vi "Disabled.vi"(7 "Robot Mode":T2, 10 "Match Info":T1={"Autonomous Elapsed Seconds"=0.0, "TeleOp Elapsed Seconds"=0.0, "Disabled Elapsed Seconds"=0.0, "Visited Autonomous"=FALSE, "Visited TeleOp"=FALSE, "Visited Disabled"=FALSE, "Autonomous Settings"={"Autonomous Style"=enum."Independent", "VI Refnum"=refnum}}, 11 "Call Context":T3) -> ()   [LabVIEW 2015]
doc: "This VI is called each time a disabled packet is received from the DS. It is often used to prepare for the next robot mode, to calibrate sensors, etc."
uses:
  <vilib>/Rock Robotics/WPI/DriverStation/WPI_DriverStationDerivedRobotMode.ctl
  <vilib>/Rock Robotics/WPI/DriverStation/WPI_DriverStationRobotMode2.ctl
  <vilib>/Rock Robotics/WPI/DriverStation/WPI_DriverStationMatch Info.ctl
  <vilib>/Rock Robotics/WPI/Utilities/WPI_GetSetVariantRefNum.vi
  Robot Global Data.vi
  Moose Code/Auto_Conf.vi
  <vilib>/Rock Robotics/Network Tables/NT Write Boolean.vi
  <vilib>/Rock Robotics/Network Tables/NT Write Number.vi
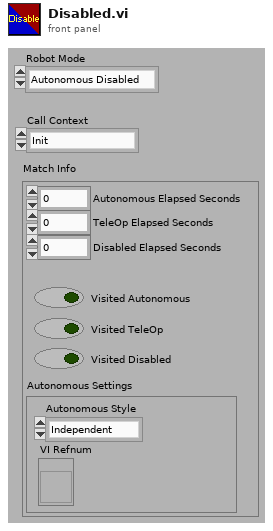
[diagram p1: front panel]
types:
  T1 = typedef "WPI_DriverStationMatch Info.ctl" = cluster{"Autonomous Elapsed Seconds":dbl, "TeleOp Elapsed Seconds":dbl, "Disabled Elapsed Seconds":dbl, "Visited Autonomous":bool, "Visited TeleOp":bool, "Visited Disabled":bool, "Autonomous Settings":cluster{"Autonomous Style":enum16{"Iterative", "Independent"}, "VI Refnum":refnum<vi>}}
  T2 = typedef "WPI_DriverStationRobotMode2.ctl" = enum16{"Autonomous Disabled", "Autonomous Enabled", "Teleop Disabled", "Teleop Enabled", "Disconnected", "Finish", "Test Disabled", "Test Enabled", "Emergency Stopped"}
  T3 = typedef "WPI_DriverStationDerivedRobotMode.ctl" = enum16{"Init", "Execute", "Stop"}
  T4 = typedef "WPI_JoystickDevRef.ctl" = cluster{"Device":T5}
  T5 = typedef "WPI_JoystickDeviceEnum.ctl" = enum16{"USB 0", "USB 1", "USB 2", "USB 3", "USB 4", "USB 5"}
  T6 = cluster{"TopLeft":bool, "TopCenter":bool, "TopRight":bool, "MiddleRight":bool, "MiddleLeft":bool, "MiddleCenter":bool, "BottomRight":bool, "BottomLeft":bool, "BottomCenter":bool, "Top":bool, "Middle":bool, "Bottom":bool, "Left":bool, "Center":bool, "Right":bool}
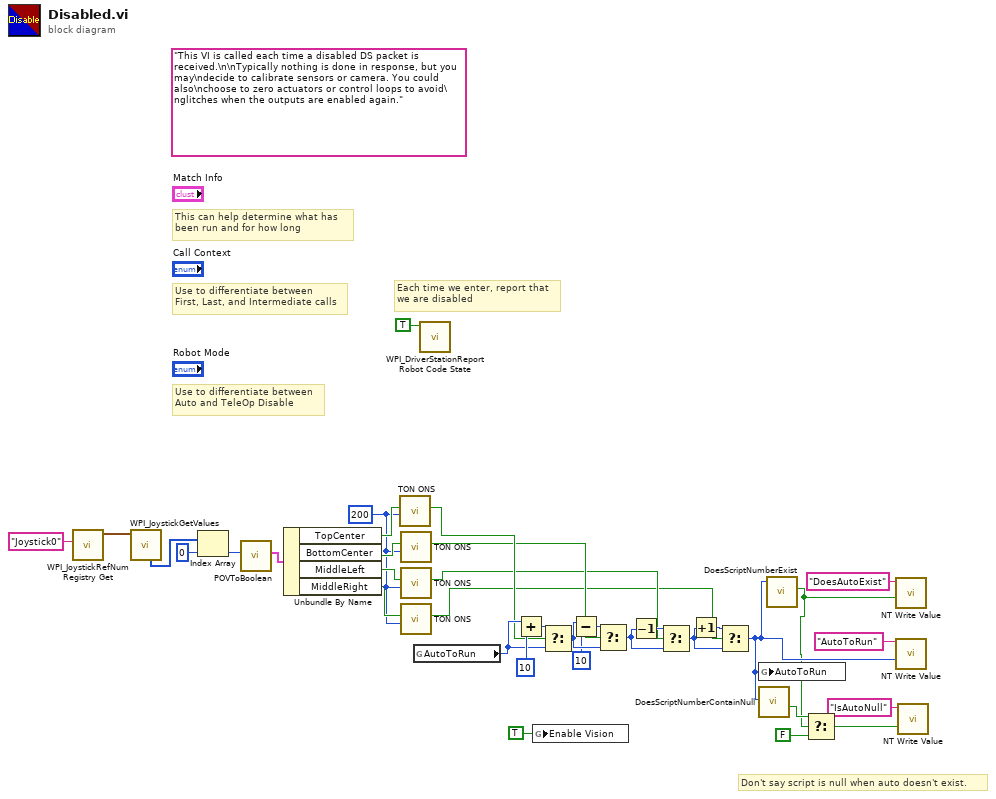
[diagram p0: block diagram]
diagram:
  w8 = u32 200 ("Delay (ms)")
  (unwired) "This VI is called each time a disabled DS packet is received.\n\nTypically nothing is done in response, but you may\ndecide to calibrate sensors or camera. You could also\nchoose to zero actuators or control loops to avoid\nglitches when the outputs are enabled again."
  # "Don't say script is null when auto doesn't exist."
  # "Each time we enter, report that\nwe are disabled"
  # "Use to differentiate between\nFirst, Last, and Intermediate calls"
  # "This can help determine what has\nbeen run and for how long"
  # "Use to differentiate between\nAuto and TeleOp Disable"
  n1 = call <vilib>:"WPI_JoystickRefNum Registry Get.vi"("refnum name"="Joystick0") -> ("JoystickDevRef"=w17:T4)  [unwired: 9 in, 1 out]
  n2 = call <vilib>:"WPI_JoystickGetValues.vi"("JoystickDevRef"=w17) -> ("POVs"=w31:i16[])  [unwired: 6 in, 4 out]
  n3 = Index Array(array=w31, index=0) -> (element=w29:i16)
  n4 = call "POVToBoolean.vi"("Input"=w29) -> ("Output"=w28:T6)  [unwired: 10 in]
  n5 = Unbundle By Name(w28) -> ("TopCenter"=w16:bool, "BottomCenter"=w14:bool, "MiddleLeft"=w12:bool, "MiddleRight"=w10:bool)
  n6 = call "TON ONS.vi"("Delay (ms)"=w8, "Input"=w16) -> ("Output 2"=w15:bool)  [unwired: 9 in]
  n7 = call "TON ONS.vi"("Delay (ms)"=w8, "Input"=w14) -> ("Output 2"=w13:bool)  [unwired: 9 in]
  n8 = call "TON ONS.vi"("Delay (ms)"=w8, "Input"=w12) -> ("Output 2"=w11:bool)  [unwired: 9 in]
  n9 = call "TON ONS.vi"("Delay (ms)"=w8, "Input"=w10) -> ("Output 2"=w9:bool)  [unwired: 9 in]
  n10 = global read "Auto_Conf.vi" "AutoToRun"() -> (w19:u8)
  n11 = call <vilib>:"WPI_DriverStationReport Robot Code State.vi"("Disabled"=TRUE ("Autonomous")) -> ()  [unwired: 10 in, 1 out]
  n12 = Add(x=w19, y=u8 10) -> (x+y=w21:u8)
  n13 = global write "Robot Global Data.vi" "Enable Vision"(TRUE ("Enable Vision")) -> ()
  n14 = Select(t=w21, s=w15, f=w19) -> (s? t:f=w26:u8)
  n15 = Subtract(x=w26, y=u8 10) -> (x-y=w27:u8)
  n16 = Select(t=w27, s=w13, f=w26) -> (s? t:f=w18:u8)
  n17 = Decrement(x=w18) -> (x-1=w22:u8)
  n18 = Select(t=w22, s=w11, f=w18) -> (s? t:f=w24:u8)
  n19 = Increment(x=w24) -> (x+1=w23:u8)
  n20 = Select(t=w23, s=w9, f=w24) -> (s? t:f=w7:u8)
  n21 = global write "Auto_Conf.vi" "AutoToRun"(w7) -> ()
  n22 = call "DoesScriptNumberContainNull.vi"("Script Index"=w7) -> ("Contains Null?"=w5:bool)  [unwired: 10 in]
  n23 = call "DoesScriptNumberExist.vi"("Script Index"=w7) -> ("file or folder exists?"=w2:bool)  [unwired: 10 in]
  n24 = Select(t=w5, s=w2, f=FALSE) -> (s? t:f=w4:bool)
  n25 = call-poly <vilib>:"NT Write Value.vi"("Boolean"=w2, "Name"="DoesAutoExist") -> ()  [unwired: 9 in, 1 out]
  n26 = call-poly <vilib>:"NT Write Value.vi"("Numeric"=w7, "Name"="AutoToRun") -> ()  [unwired: 9 in, 1 out]
  n27 = call-poly <vilib>:"NT Write Value.vi"("Boolean"=w4, "Name"="IsAutoNull") -> ()  [unwired: 9 in, 1 out]
